vi "Copy Image To Output.vi"(8 "Error In":errorcluster, 10 "Paths to copy":path[](array[path]), 11 "Directory to copy to":path) -> (0 "Error Out":errorcluster)   [LabVIEW 2014, in "i3-docs.lvlib"]
uses:
  i3-docs.lvlib
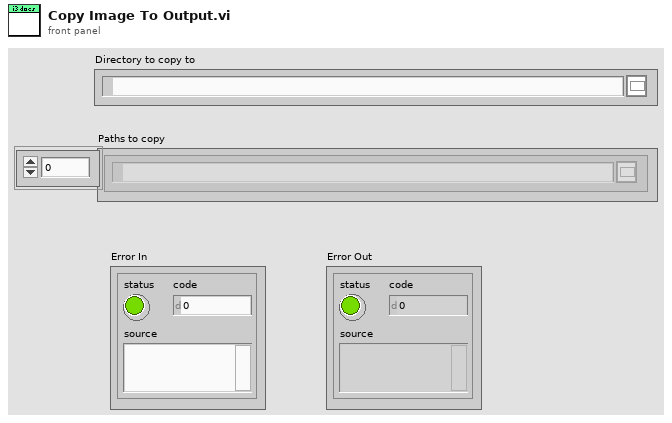
[diagram p1: front panel]
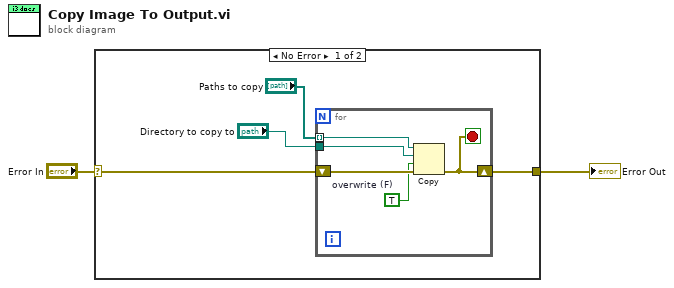
[diagram p0: block diagram]
diagram:
  n1 = case shown="No Error" "Error In" {
    selector: "Error In" -> [w3 w12]
    tunnel: [w6 w12] -> w2
    frame No Error {
      n2 = for {
        tunnel: "Paths to copy" -> [w10] mode=indexing
        shift-right: [w8] -> w6
        shift-left: w3 -> [w11]
        tunnel: "Directory to copy to" -> [w7]
        stop <- w8 stop-if-true
        w9 = TRUE  # overwrite (F)
        n3 = Copy(8:w11, 9:w9, 10:w7, 11:w10) -> (0:w8:errorcluster)  [unwired: 1 in, 2 out]
      }
    }
    frame Error {
    }
  }
  "Error Out" <- w2
